vi "Convert Decay Fit Options v1 to v2.vi"(1 "Decay Fit Options v1":T1 {"Offset Resolution" min=0.0; "Period" min=0.0; "Min Decay Percentile" min=0.0 max=1.0; "Max Decay Percentile" min=0.0 max=100.0}) -> (0 "Decay Fit Options v2":T8={"Show Fit Residuals"=TRUE, "Fit Model"=enum."1-Exponential", "Residual Type"=enum."Standard", "Max Decay Percentile"=0.0, "Min Decay Percentile"=0.0, "Show Full Decay"=TRUE, "Weights"=enum."Unweighted", "Fitting Method"=enum."Least Square", "Compute Parameter Uncertainties"=TRUE, "Periodic Boundaries"=TRUE, "Model Calculation"=enum."Simulation", "Period"=1.2500000000000001e-08, "Termination Criteria"={"Max Iterations"=0, "Max Function Calls"=0, "Max Time"=1000.0, "Function Tolerance"=1e-06, "Parameter Tolerance"=1e-06, "Gradient Tolerance"=0.0, "Min Lambda"=1e-06, "Max Lambda"=1e-06, "Initial Tick Count"=0}, "Offset Resolution"=1.2500000000000001e-08, "Use Local IRF"=TRUE, "Fitting Algorithm"=enum."Levenberg-Marquardt"} {"Offset Resolution" min=0.0; "Period" min=0.0; "Min Decay Percentile" min=0.0 max=1.0; "Max Decay Percentile" min=0.0 max=1.0})   [LabVIEW 2021, in "Fits.lvlib"]
uses:
  Fits.lvlib
  Decay Fit Options v2.ctl
  Decay Convolution/Decay Model.ctl
  Residual Type.ctl
  Fit Weights Type.ctl
  Non-linear Fitting Method v2.ctl
  Fit Calculation Method.ctl
  Non-linear Fitting Algorithm.ctl
  Decay Fit Options v1.ctl
  Non-linear Fitting Method v1.ctl
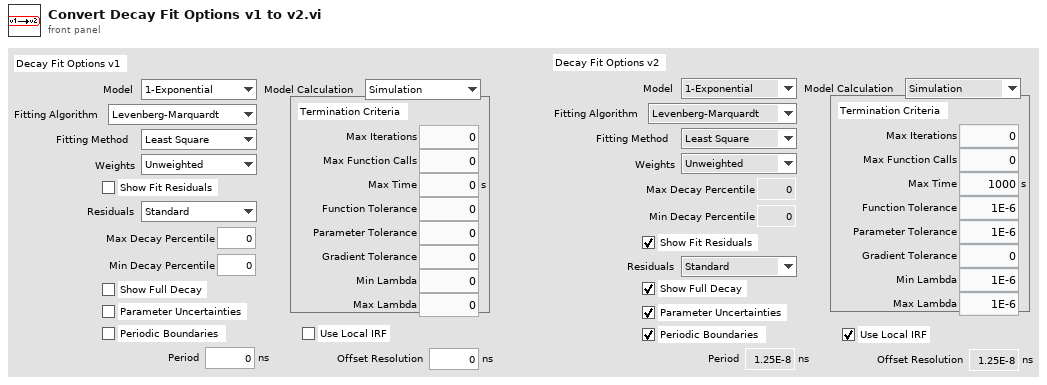
[diagram p1: front panel]
types:
  T1 = typedef "Fits.lvlib/Decay Fit Options v1.ctl" = cluster{"Show Fit Residuals":bool, "Fit Model":T2, "Residual Type":T3, "Max Decay Percentile":dbl, "Min Decay Percentile":dbl, "Show Full Decay":bool, "Weights":T4, "Fitting Method":T5, "Compute Parameter Uncertainties":bool, "Periodic Boundaries":bool, "Model Calculation":T6, "Period":dbl[unit], "Termination Criteria":cluster{"Max Iterations":i32, "Max Function Calls":i32, "Max Time":dbl[unit], "Function Tolerance":dbl, "Parameter Tolerance":dbl, "Gradient Tolerance":dbl, "Min Lambda":dbl, "Max Lambda":dbl, "Initial Tick Count":u32}, "Offset Resolution":dbl[unit], "Use Local IRF":bool, "Fitting Algorithm":T7}
  T2 = typedef "Fits.lvlib/Decay Model.ctl" = enum16{"1-Exponential", "2-Exponentials"}
  T3 = typedef "Fits.lvlib/Residual Type.ctl" = enum16{"Standard", "Normalized", "Reduced"}
  T4 = typedef "Fits.lvlib/Fit Weights Type.ctl" = enum16{"Unweighted", "1/Variance", "Best of All"}
  T5 = typedef "Fits.lvlib/Non-linear Fitting Method v1.ctl" = enum16{"Least Square", "Least Absolute Residual", "Bisquare", "-", "Best of All"}
  T6 = typedef "Fits.lvlib/Fit Calculation Method.ctl" = enum16{"Simulation", "Convolution", "Integration"}
  T7 = typedef "Fits.lvlib/Non-linear Fitting Algorithm.ctl" = enum16{"Levenberg-Marquardt", "Trust-Region Dogleg"}
  T8 = typedef "Fits.lvlib/Decay Fit Options v2.ctl" = cluster{"Show Fit Residuals":bool, "Fit Model":T2, "Residual Type":T3, "Max Decay Percentile":dbl, "Min Decay Percentile":dbl, "Show Full Decay":bool, "Weights":T4, "Fitting Method":T9, "Compute Parameter Uncertainties":bool, "Periodic Boundaries":bool, "Model Calculation":T6, "Period":dbl[unit], "Termination Criteria":cluster{"Max Iterations":i32, "Max Function Calls":i32, "Max Time":dbl[unit], "Function Tolerance":dbl, "Parameter Tolerance":dbl, "Gradient Tolerance":dbl, "Min Lambda":dbl, "Max Lambda":dbl, "Initial Tick Count":u32}, "Offset Resolution":dbl[unit], "Use Local IRF":bool, "Fitting Algorithm":T7}
  T9 = typedef "Fits.lvlib/Non-linear Fitting Method v2.ctl" = enum16{"Least Square", "Least Absolute Residual", "Bisquare", "MLE", "-", "Best of All"}
  T10 = cluster{"Max Iterations":i32, "Max Function Calls":i32, "Max Time":dbl[unit], "Function Tolerance":dbl, "Parameter Tolerance":dbl, "Gradient Tolerance":dbl, "Min Lambda":dbl, "Max Lambda":dbl, "Initial Tick Count":u32}
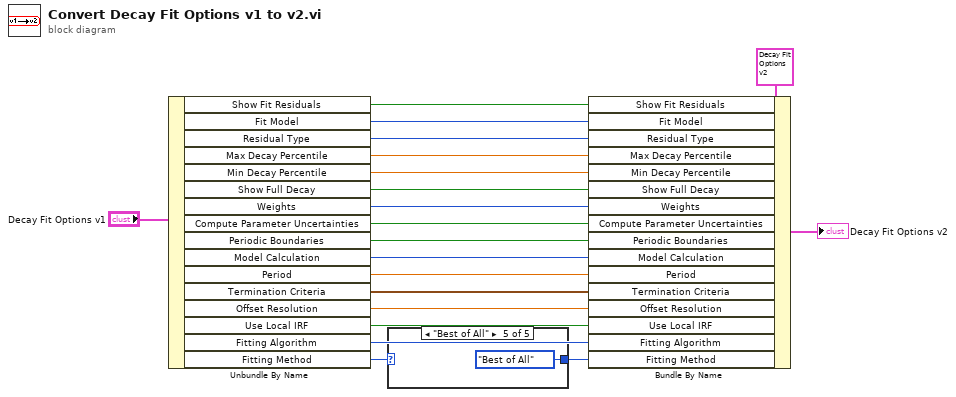
[diagram p0: block diagram]
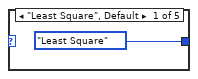
[diagram p2: hidden frame]
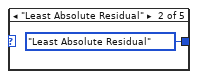
[diagram p3: hidden frame]
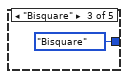
[diagram p4: hidden frame]
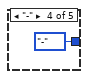
[diagram p5: hidden frame]
diagram:
  n1 = Unbundle By Name("Decay Fit Options v1") -> ("Show Fit Residuals"=w17:bool, "Fit Model"=w16:T2, "Residual Type"=w15:T3, "Max Decay Percentile"=w14:dbl, "Min Decay Percentile"=w13:dbl, "Show Full Decay"=w12:bool, "Weights"=w11:T4, "Compute Parameter Uncertainties"=w10:bool, "Periodic Boundaries"=w9:bool, "Model Calculation"=w8:T6, "Period"=w7:dbl[unit], "Termination Criteria"=w5:T10, "Offset Resolution"=w6:dbl[unit], "Use Local IRF"=w4:bool, "Fitting Algorithm"=w3:T7, "Fitting Method"=w2:T5)
  n2 = case shown="\"Best of All\"" w2 {
    tunnel: [Non-linear_Fitting_Method_v2."Least Square" ("Fitting Method") Non-linear_Fitting_Method_v2."Least Absolute Residual" ("Fitting Method") Non-linear_Fitting_Method_v2."Bisquare" ("Fitting Method") Non-linear_Fitting_Method_v2."-" ("Fitting Method") Non-linear_Fitting_Method_v2."Best of All" ("Fitting Method")] -> w1
    frame "Least Square", Default {
    }
    frame "Least Absolute Residual" {
    }
    frame "Bisquare" {
    }
    frame "-" {
    }
    frame "Best of All" {
    }
  }
  n3 = Bundle By Name(cluster=T8 {"Show Fit Residuals"=TRUE, "Fit Model"=enum."1-Exponential", "Residual Type"=enum."Standard", "Max Decay Percentile"=0.0, "Min Decay Percentile"=0.0, "Show Full Decay"=TRUE, "Weights"=enum."Unweighted", "Fitting Method"=enum."Least Square", "Compute Parameter Uncertainties"=TRUE, "Periodic Boundaries"=TRUE, "Model Calculation"=enum."Simulation", "Period"=1.2500000000000001e-08, "Termination Criteria"={"Max Iterations"=0, "Max Function Calls"=0, "Max Time"=1000.0, "Function Tolerance"=1e-06, "Parameter Tolerance"=1e-06, "Gradient Tolerance"=0.0, "Min Lambda"=1e-06, "Max Lambda"=1e-06, "Initial Tick Count"=0}, "Offset Resolution"=1.2500000000000001e-08, "Use Local IRF"=TRUE, "Fitting Algorithm"=enum."Levenberg-Marquardt"} ("Decay Fit Options v2"), "Show Fit Residuals"=w17, "Fit Model"=w16, "Residual Type"=w15, "Max Decay Percentile"=w14, "Min Decay Percentile"=w13, "Show Full Decay"=w12, "Weights"=w11, "Compute Parameter Uncertainties"=w10, "Periodic Boundaries"=w9, "Model Calculation"=w8, "Period"=w7, "Termination Criteria"=w5, "Offset Resolution"=w6, "Use Local IRF"=w4, "Fitting Algorithm"=w3, "Fitting Method"=w1) -> (→"Decay Fit Options v2":T8)
